vi "hidSPD Get Heatsink Tempratures From Reports.vi"(10 "spd Reports in":T1[](array[typedef])) -> (2 "Heatsink Tempratures":sgl[](array[numeric]))   [LabVIEW 2018, in "hidSPDLibForLabView.lvlib"]
uses:
  hidSPDLibForLabView.lvlib
  hidSPD Controls/hidSPD Simple Report.ctl
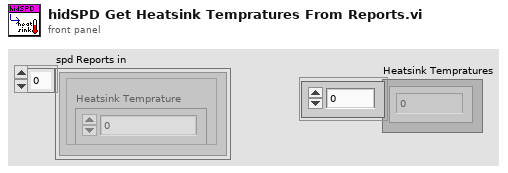
[diagram p1: front panel]
types:
  T1 = typedef "hidSPDLibForLabView.lvlib/hidSPD Simple Report.ctl" = cluster{"Heatsink Temprature":sgl, "Diod Temprature":sgl, "TEC-voltage":sgl, "Diod Bias":sgl, "RF Power":sgl, "Thrm_used":sgl, "Thrm_end":sgl, "Thrm_error":sgl, "stableI":sgl, "pid_error":sgl, "strobe code used":u16, "SPD number":u8, "SPD ready":u8, "status SPD":u32}
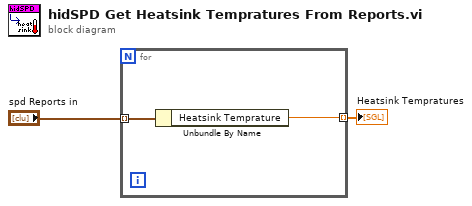
[diagram p0: block diagram]
diagram:
  n1 = for {
    tunnel: "spd Reports in" -> [w4] mode=indexing
    tunnel: [w3] -> w1 mode=indexing
    n2 = Unbundle By Name(w4) -> ("Heatsink Temprature"=w3:sgl)
  }
  "Heatsink Tempratures" <- w1
